vi "Create Chart.vi"() -> ()   [LabVIEW 2016, in "CML UI.lvlib" / "Circular Cue Helper.lvlib"]
doc: "This is a test VI using Pie Chart subVI to show what the chart looks like."
uses:
  Circular Cue Helper.lvlib
panel:
  out "Picture":picture
  in  "Test Value":cluster{"Label":string, "Value":dbl}[](array[cluster])=[{"Label"="This", "Value"=23.0}, {"Label"="is", "Value"=13.0}, {"Label"="only", "Value"=36.0}, {"Label"="a", "Value"=7.0}, {"Label"="test", "Value"=21.0}]
  # "Overview: This is a test VI using Pie Chart subVI to show what the chart looks like.\nRequirements: LabVIEW 2012 (or compatible)\nInstructions:\n1. Specify the Labels and Values in Test Value cluster.\n2. Run this VI and a pie chart with legend is generated and displayed.\n3. Open the Pie Chart 2012 to show the details."
  # "Test Chart"
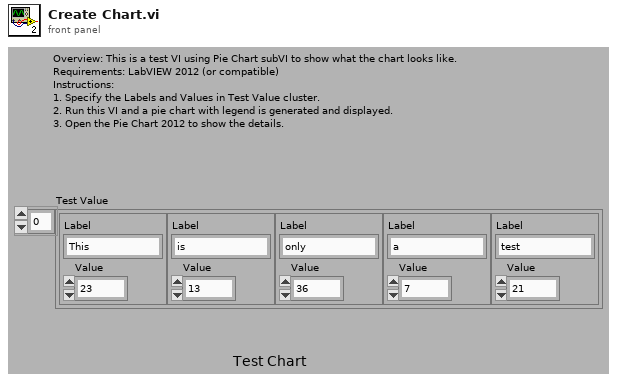
[diagram p1: front panel]
types:
  T1 = typedef "LVBoundsTypeDef.ctl" = cluster{"Width":u32, "Height":u32}
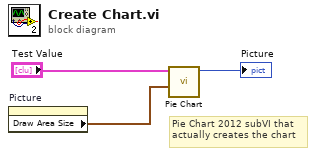
[diagram p0: block diagram]
diagram:
  # "Pie Chart 2012 subVI that \nactually creates the chart"
  n1 = property on="Picture" class="Pict"() -> ("Draw Area Size"=w1:T1)  [unwired: 2 in, 2 out]
  n2 = call "Pie Chart.vi"("Draw Area Size"=w1, "Array"="Test Value") -> ("Picture"=→"Picture":picture)  [unwired: 9 in]
